vi "NMEA_ParseMessage-GPVTG.vi"(9 "Error In":errorcluster, 10 "$GPVTG-message_IN":string) -> (1 "Error Out":errorcluster, 2 "$GPVTG-message_OUT":T1={"True Course over Ground"=0.0, "Magnetic Course over Ground"=0.0, "Speed over Ground in knots"=0.0, "Speed over Ground in km/h"=1.0, "Mode"=""} {"Speed over Ground in km/h" format="%.02f [km/h]"; "Speed over Ground in knots" format="%.02f [kts]"; "Magnetic Course over Ground" format="%.02f [deg]"; "True Course over Ground" format="%.02f [deg]"})   [LabVIEW 2016, in "环境动力监测库.lvlib" / "AIRMAR WeatherCaster.lvlib"]
doc: "<B>GPVTG</B>\nTrack Made Good and Ground Speed"
uses:
  AIRMAR WeatherCaster.lvlib
  NMEA_GPVTG-data.ctl
  NMEA_Mode.ctl
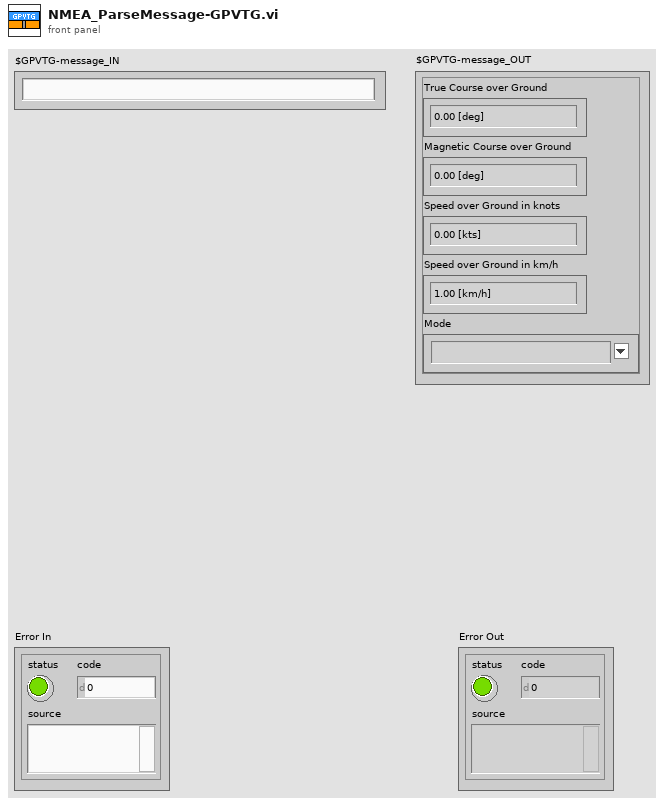
[diagram p1: front panel]
types:
  T1 = typedef "环境动力监测库.lvlib/AIRMAR WeatherCaster.lvlib/NMEA_GPVTG-data.ctl" = cluster{"True Course over Ground":dbl, "Magnetic Course over Ground":dbl, "Speed over Ground in knots":dbl, "Speed over Ground in km/h":dbl, "Mode":T2}
  T2 = typedef "环境动力监测库.lvlib/AIRMAR WeatherCaster.lvlib/NMEA_Mode.ctl" = string
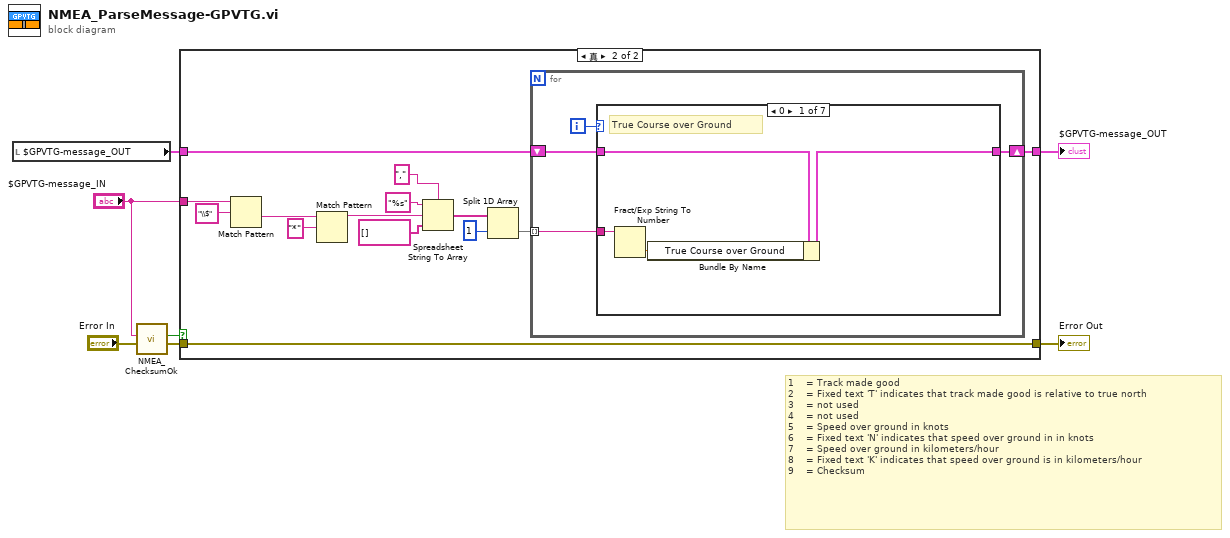
[diagram p0: block diagram]
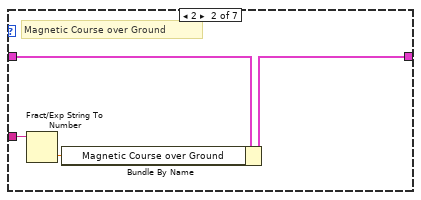
[diagram p3: hidden frame]
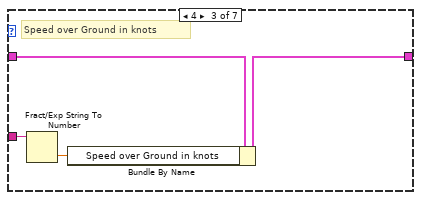
[diagram p4: hidden frame]
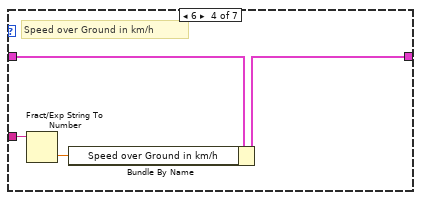
[diagram p5: hidden frame]
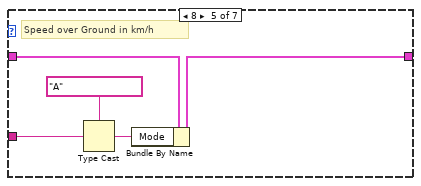
[diagram p6: hidden frame]
diagram:
  # "1    = Track made good\n2    = Fixed text 'T' indicates that track made good is relative to true north\n3    = not used\n4    = not used\n5    = Speed over ground in knots\n6    = Fixed text 'N' indicates that speed over ground in in knots\n7    = Speed over ground in kilometers/hour\n8    = Fixed text 'K' indicates that speed over ground is in kilometers/hour\n9    = Checksum"
  n1 = local read "$GPVTG-message_OUT"() -> (w7:T1)
  n2 = call "NMEA_ChecksumOk.vi"("Error In"="Error In", "Sentence"="$GPVTG-message_IN") -> ("Error Out"=w1:errorcluster, "CheckSumOk?"=w4:bool)  [unwired: 8 in]
  n3 = case shown="真" w4 {
    tunnel: w7 -> [w9 w18]
    tunnel: [w9 w17] -> w6
    tunnel: "$GPVTG-message_IN" -> [_ w15]
    tunnel: w1 -> [w8 w10]
    tunnel: [w8 w10] -> w3
    frame False {
    }
    frame True {
      n4 = Match Pattern(string=w15, regular expression="\\$") -> (after substring=w14:string)  [unwired: 1 in, 3 out]
      n5 = Match Pattern(string=w14, regular expression="*") -> (before substring=w22:string)  [unwired: 1 in, 3 out]
      n6 = Spreadsheet String To Array(delimiter (Tab)=",", format string="%s", spreadsheet string=w22, array type (2D Dbl)=string[] []) -> (array=w12:string[])
      n7 = Split 1D Array(array=w12, index=1) -> (second subarray=w13:string[])  [unwired: 1 out]
      n8 = for {
        tunnel: w13 -> [w24] mode=indexing
        shift-right: [w26] -> w17
        shift-left: w18 -> [w27]
        i -> [w25]
        n9 = case shown="0" w25 {
          tunnel: w27 -> [w31 w35 w39 w43 w48 w49 w50]
          tunnel: [w30 w34 w38 w42 w47 w49 w50] -> w26
          tunnel: w24 -> [w29 w33 w37 w41 w45 _ _]
          frame 0 {
            # "True Course over Ground"
            n10 = Fract/Exp String To Number(string=w29) -> (number=w28:dbl)  [unwired: 3 in, 1 out]
            n11 = Bundle By Name(cluster=w31, "True Course over Ground"=w28) -> (w30:T1)
          }
          frame 2 {
            # "Magnetic Course over Ground"
            n12 = Fract/Exp String To Number(string=w33) -> (number=w32:dbl)  [unwired: 3 in, 1 out]
            n13 = Bundle By Name(cluster=w35, "Magnetic Course over Ground"=w32) -> (w34:T1)
          }
          frame 4 {
            # "Speed over Ground in knots"
            n14 = Fract/Exp String To Number(string=w37) -> (number=w36:dbl)  [unwired: 3 in, 1 out]
            n15 = Bundle By Name(cluster=w39, "Speed over Ground in knots"=w36) -> (w38:T1)
          }
          frame 6 {
            # "Speed over Ground in km/h"
            n16 = Fract/Exp String To Number(string=w41) -> (number=w40:dbl)  [unwired: 3 in, 1 out]
            n17 = Bundle By Name(cluster=w43, "Speed over Ground in km/h"=w40) -> (w42:T1)
          }
          frame 8 {
            # "Speed over Ground in km/h"
            n18 = Type Cast(type=T2 "A" ("Mode"), x=w45) -> (*(type *) &x=w44:T2)
            n19 = Bundle By Name(cluster=w48, "Mode"=w44) -> (w47:T1)
          }
          frame 1, 3, 5, 7 {
            # "[1] - True course over ground indicator (always 'T')\n[3] - Magnetic course over ground indicator (always 'M')\n[5] - Speed over ground in knots indicator (always 'N')\n[7] - Speed over ground in km/h indicator (always 'K')"
          }
          frame Default {
          }
        }
      }
    }
  }
  "$GPVTG-message_OUT" <- w6
  "Error Out" <- w3
